vi "Get 1D Array Double Complex.vi"(5 "use temporary file? (F)":bool, 7 "data type of variable":cdb[](array[numeric]), 8 "error in":errorcluster, 10 "variable name":string, 11 "GOLPI ref. in":T1={"pipe handle"={"lv_proc.dll file path"=path "", "process instance handle"=[], "debug mode"=FALSE, "debug data"=[]}, "fast read timeout [ms]"=500, "fast read settle time [ms]"=10, "fast read to multiple [ms]"=1, "max elements per input line"=100, "slow read timeout [ms]"=5000, "stdin double format specifier"="%_16e", "max elements per stdout output column"=100, "console mode bitstream"=FALSE, "bitstream first read timeout [ms]"=1000, "bitstream read timeout [ms]"=50, "struct transfer possible"=FALSE, "matlab mode"=FALSE, "var pipe write timeout [ms]"=5000, "variable pipe mode"=FALSE, "variable pipe buffer size [Bytes]"=10000000, "variable pipe block size [Bytes]"=1000000} {"variable pipe block size [Bytes]" format="%.0p"; "variable pipe buffer size [Bytes]" format="%.0p"}) -> (0 "error out":errorcluster, 2 "value":cdb[](array[numeric]) format="%.2f", 3 "GOLPI ref. out":T1={"pipe handle"={"lv_proc.dll file path"=path "", "process instance handle"=[], "debug mode"=FALSE, "debug data"=[]}, "fast read timeout [ms]"=500, "fast read settle time [ms]"=10, "fast read to multiple [ms]"=1, "max elements per input line"=100, "slow read timeout [ms]"=5000, "stdin double format specifier"="%_16e", "max elements per stdout output column"=100, "console mode bitstream"=FALSE, "bitstream first read timeout [ms]"=1000, "bitstream read timeout [ms]"=50, "struct transfer possible"=FALSE, "matlab mode"=FALSE, "var pipe write timeout [ms]"=5000, "variable pipe mode"=FALSE, "variable pipe buffer size [Bytes]"=10000000, "variable pipe block size [Bytes]"=1000000} {"variable pipe block size [Bytes]" format="%.0p"; "variable pipe buffer size [Bytes]" format="%.0p"})   [LabVIEW 2020, in "GOLPI library.lvlib"]
doc: "Part of polymorph Get Variable.vi"
uses:
  GOLPI library.lvlib
  Public/GOLPI reference Type Def.ctl
  LV Process source distribution/Pipe Handle.ctl
  Type Definitions/Bitstream Data Type.ctl
  Type Definitions/Custom Error Codes Enum Type Def.vi
  LV Process source distribution/LV Process library.lvlib
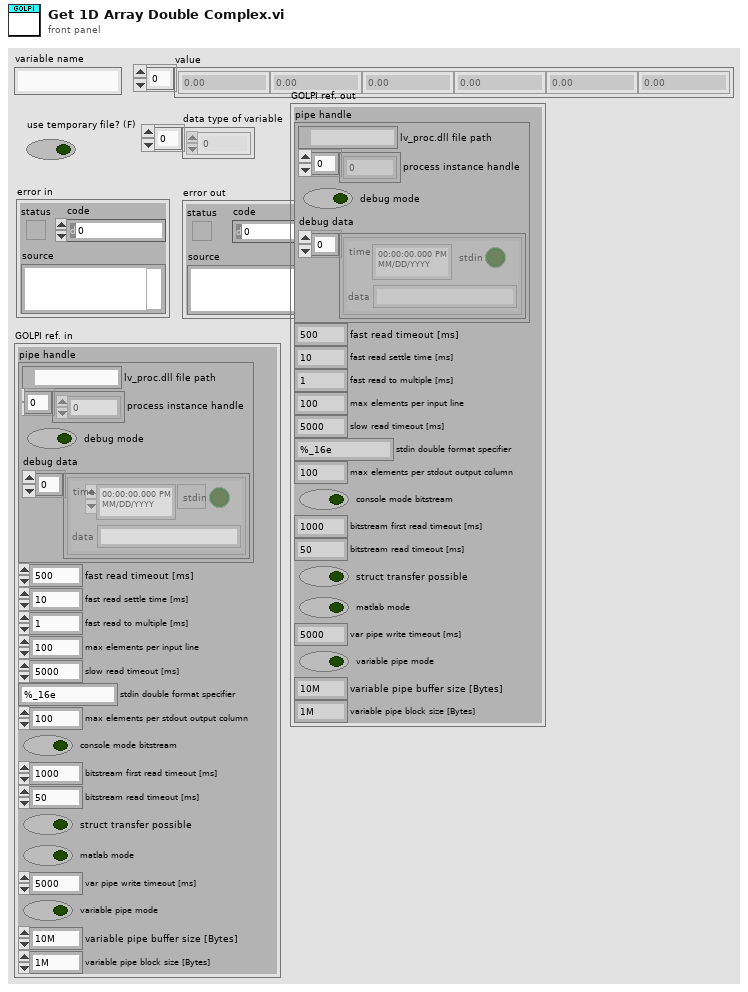
[diagram p1: front panel]
types:
  T1 = typedef "GOLPI library.lvlib/GOLPI reference Type Def.ctl" = cluster{"pipe handle":T2, "fast read timeout [ms]":u32, "fast read settle time [ms]":u32, "fast read to multiple [ms]":u32, "max elements per input line":u32, "slow read timeout [ms]":u32, "stdin double format specifier":string, "max elements per stdout output column":u32, "console mode bitstream":bool, "bitstream first read timeout [ms]":u32, "bitstream read timeout [ms]":u32, "struct transfer possible":bool, "matlab mode":bool, "var pipe write timeout [ms]":u32, "variable pipe mode":bool, "variable pipe buffer size [Bytes]":u32, "variable pipe block size [Bytes]":u32}
  T2 = typedef "LV Process library.lvlib/Pipe Handle.ctl" = cluster{"lv_proc.dll file path":path, "process instance handle":u32[], "debug mode":bool, "debug data":cluster{"time":timestamp, "stdin":bool, "data":string}[]}
  T3 = typedef "GOLPI library.lvlib/Custom Error Codes Enum Type Def.vi" = enum16{"no error", "00 working directory PAR1 missing", "01 octave binary PAR1 missing", "02 octave report error PAR1", "03 empty output last cmd PAR1", "04 missing temporary file PAR1", "05 pwd PAR 1 not exist", "06 oct package not installed", "07 octave default binary missing", "10 var PAR1 not string, vect", "11 var PAR1 not num, scal, ~compl", "12 var PAR1 not num, scal, compl", "13 var PAR1 not num, vect, ~compl", "14 var PAR1 not num, vect, compl", "15 var PAR1 not num, mat, ~compl", "16 var PAR1 not num, mat, ~compl", "30 read timeout", "60 bitstream transport failed", "61 bitstream decode error PAR1", "62 bitstream cannot be set", "70 struct transfer not possible", "80 struct: cluster elem. PAR1 not implem.", "81 struct: structure field PAR1 not implem.", "82 struct: size mismatch of PAR1", "83 struct: type mismatch of PAR1", "98 internal error", "99 not finished", "90 Not supported in Matlab mode", "91 Matlab variable transfer error", "92 Matlab Script Error"}
  T4 = typedef "GOLPI library.lvlib/Bitstream Data Type.ctl" = enum16{"dummy", "int", "uint", "float", "complex", "str", "real numeric"}
  T5 = typedef "GOLPI library.lvlib/Transfer Mode.ctl" = enum16{"Matlab", "stdio", "temp file", "bitstream", "pipe"}
  T6 = typedef "GOLPI library.lvlib/Bitstream Data.ctl" = cluster{"double":dbl[][], "cplx double":cdb[][], "int64":i64[][], "uint64":u64[][], "str":string[], "data type":T4}
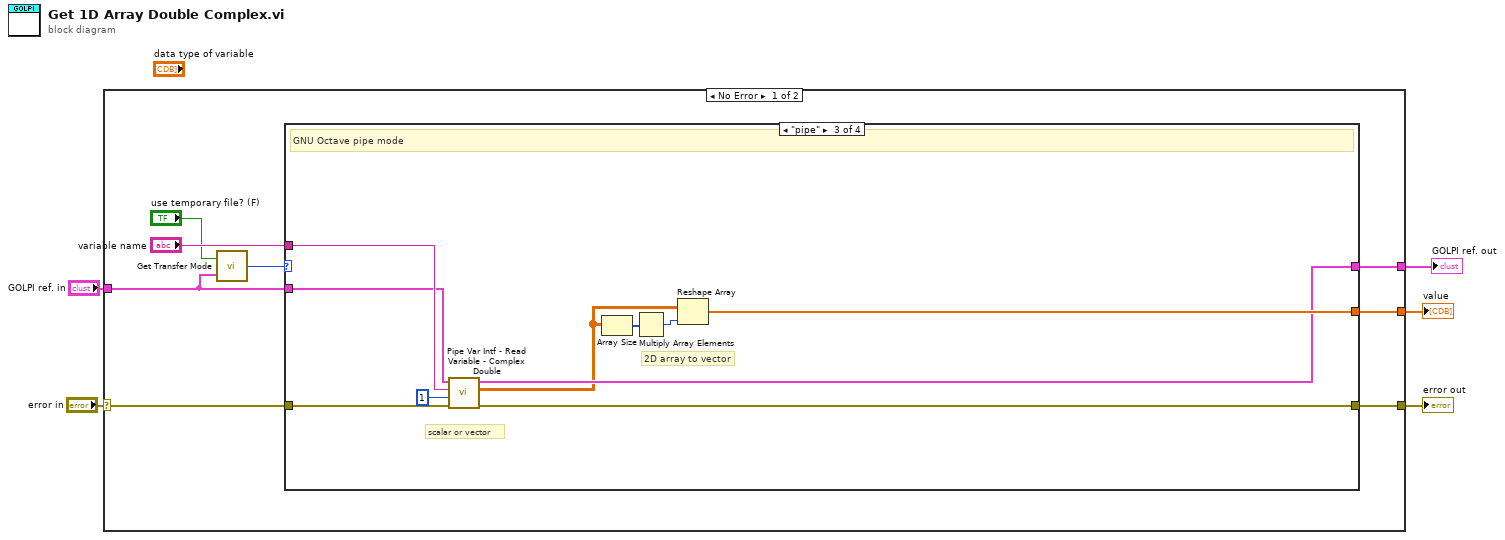
[diagram p0: block diagram]
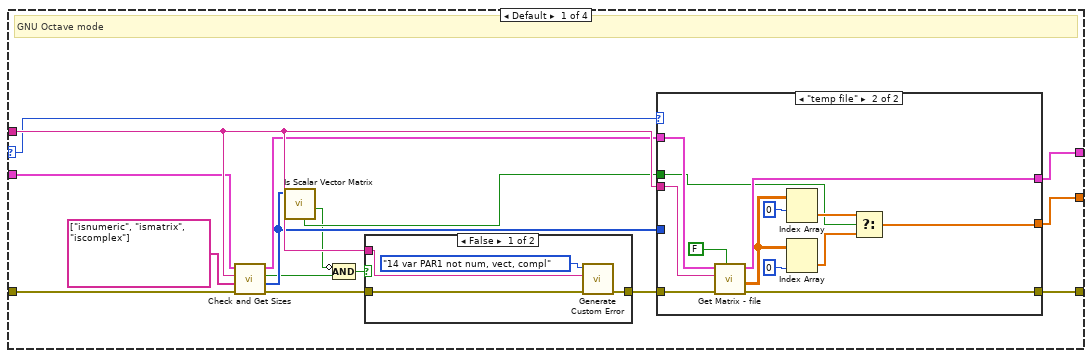
[diagram p2: hidden frame]
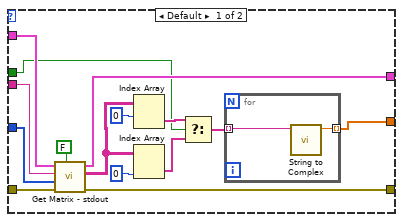
[diagram p3: hidden frame]
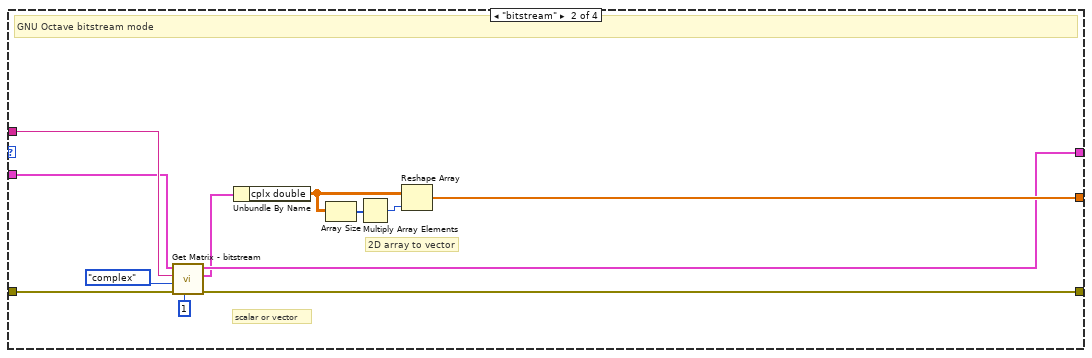
[diagram p5: hidden frame]
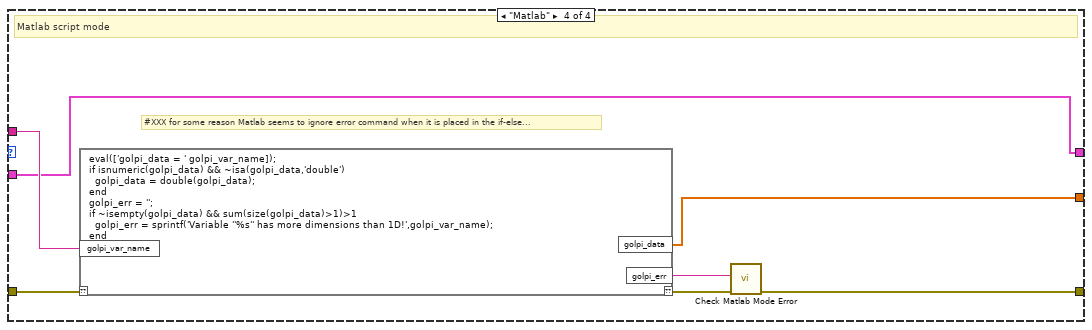
[diagram p6: hidden frame]
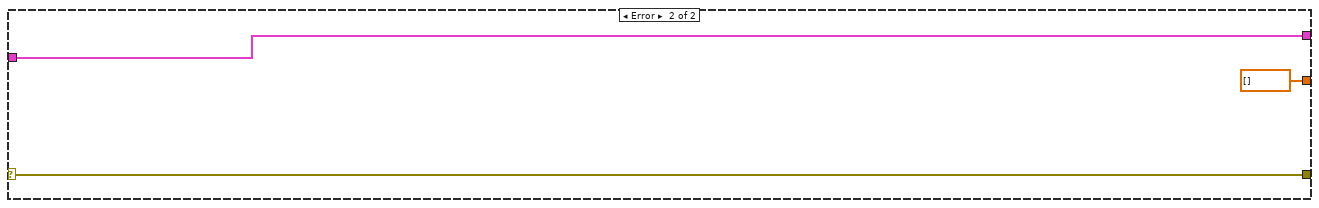
[diagram p7: hidden frame]
diagram:
  n1 = case shown="No Error" "error in" {
    selector: "error in" -> [w13 w96]
    tunnel: [w12 w96] -> w5
    tunnel: [w10 cdb[] [] ("value")] -> w3
    tunnel: "GOLPI ref. in" -> [w8 w94]
    tunnel: [w9 w94] -> w1
    frame No Error {
      n2 = call "Get Transfer Mode.vi"("GOLPI ref."=w8, "use temporary file? (F)"="use temporary file? (F)") -> ("mode"=w6:T5)
      n3 = case shown="\"pipe\"" w6 {
        selector: w6 -> [w14 _ _ _]
        tunnel: w13 -> [w29 w76 w86 w93]
        tunnel: [w28 w75 w85 w87] -> w12
        tunnel: "variable name" -> [w27 w74 w84 w92]
        tunnel: [w26 w73 w83 w90] -> w10
        tunnel: [w25 w72 w82 w91] -> w9
        tunnel: w8 -> [w24 w71 w81 w91]
        frame Default {
          # "GNU Octave mode"
          n4 = call "Check and Get Sizes.vi"("error in (no error)"=w29, "test commands"=string[] ["isnumeric", "ismatrix", "iscomplex"], "variable name"=w27, "GOLPI ref. in"=w24) -> ("error out"=w23:errorcluster, "octave sizes"=w19:i32[], "all tests OK?"=w17:bool, "GOLPI ref. out"=w21:T1)  [unwired: 4 in]
          n5 = call "Is Scalar Vector Matrix.vi"("octave sizes"=w19) -> ("is matrix?"=w15:bool, "row vector?"=w18:bool)  [unwired: 5 in, 4 out]
          n6 = Compound Arithmetic op=AND(invert w15, w17) -> (w16:bool)
          n7 = case shown="False" w16 {
            tunnel: w23 -> [w62 w64]
            tunnel: [w61 w64] -> w20
            tunnel: w27 -> [w60 _]
            frame False {
              n8 = call "Generate Custom Error.vi"("error in"=w62, "PAR1"=w60, "GOLPI error"=Custom_Error_Codes_Enum_Type_Def.vi."14 var PAR1 not num, vect, compl" ("Enum")) -> ("error out"=w61:errorcluster)  [unwired: 8 in]
            }
            frame True {
            }
          }
          n9 = case shown="\"temp file\"" w14 {
            tunnel: w21 -> [w44 w51]
            tunnel: [w43 w52] -> w25
            tunnel: w20 -> [w41 w54]
            tunnel: [w42 w53] -> w28
            tunnel: w19 -> [w40 _]
            tunnel: w18 -> [w30 w47]
            tunnel: w27 -> [w39 w48]
            tunnel: [w37 w49] -> w26
            frame Default {
              n10 = call "Get Matrix - stdout.vi"("is string?"=FALSE ("is string"), "error in (no error)"=w41, "octave sizes"=w40, "variable name"=w39, "GOLPI ref. in"=w44) -> ("error out"=w42:errorcluster, "array"=w31:string[][], "GOLPI ref. out"=w43:T1)  [unwired: 4 in]
              n11 = Index Array(array=w31, index (row)=0) -> (element=w34:string[])  [unwired: 1 in]
              n12 = Index Array(array=w31, index (col)=0 ("disabled index (col)")) -> (element=w33:string[])  [unwired: 1 in]
              n13 = Select(t=w34, s=w30, f=w33) -> (s? t:f=w32:string[])
              n14 = for {
                tunnel: w32 -> [w46] mode=indexing
                tunnel: [w45] -> w37 mode=indexing
                n15 = call "String to Complex.vi"("string"=w46) -> ("complex number"=w45:cdb)  [unwired: 10 in]
              }
            }
            frame "temp file" {
              n16 = call "Get Matrix - file.vi"("is string?"=FALSE ("is string"), "error in (no error)"=w54, "variable name"=w48, "GOLPI ref. in"=w51) -> ("error out"=w53:errorcluster, "cmplx double array"=w50:cdb[][], "GOLPI ref. out"=w52:T1)  [unwired: 3 in, 2 out]
              n17 = Index Array(array=w50, index (row)=0) -> (element=w57:cdb[])  [unwired: 1 in]
              n18 = Index Array(array=w50, index (col)=0 ("disabled index (col)")) -> (element=w56:cdb[])  [unwired: 1 in]
              n19 = Select(t=w57, s=w47, f=w56) -> (s? t:f=w49:cdb[])
            }
          }
        }
        frame "bitstream" {
          # "scalar or vector"
          # "2D array to vector"
          # "GNU Octave bitstream mode"
          n20 = call "Get Matrix - bitstream.vi"("max dimensions (0: scalar)"=1, "error in (no error)"=w76, "data type"=Bitstream_Data_Type."complex", "variable name"=w74, "GOLPI ref. in"=w71) -> ("error out"=w75:errorcluster, "data"=w65:T6, "GOLPI ref. out"=w72:T1)  [unwired: 4 in]
          n21 = Unbundle By Name(w65) -> ("cplx double"=w68:cdb[][])
          n22 = Array Size(array=w68) -> (size(s)=w67:i32[])
          n23 = Multiply Array Elements(1:w67) -> (0:w66:i32)
          n24 = Reshape Array(w68, w66) -> (w73:cdb[])
        }
        frame "pipe" {
          # "scalar or vector"
          # "2D array to vector"
          # "GNU Octave pipe mode"
          n25 = call "Pipe Var Intf - Read Variable - Complex Double.vi"("error in (no error)"=w86, "max dims (0: scalar)"=1 ("max dimensions (0: scalar)"), "variable name"=w84, "GOLPI ref. in"=w81) -> ("error out"=w85:errorcluster, "data out"=w77:cdb[][], "GOLPI ref. out"=w82:T1)  [unwired: 5 in]
          n26 = Array Size(array=w77) -> (size(s)=w79:i32[])
          n27 = Multiply Array Elements(1:w79) -> (0:w78:i32)
          n28 = Reshape Array(w77, w78) -> (w83:cdb[])
        }
        frame "Matlab" {
          # "#XXX for some reason Matlab seems to ignore error command when it is placed in the if-else..."
          # "Matlab script mode"
          n29 = script code="eval(['golpi_data = ' golpi_var_name]);\nif isnumeric(golpi_data) && ~isa(golpi_data,'double')\n  golpi_data = double(golpi_data);\nend\ngolpi_err = '';\nif ~isempty(golpi_data) && sum(size(golpi_data)>1)>1\n  golpi_err = sprintf('Variable ''%s'' has more dimensions than 1D!',golpi_var_name);\nend"("??"=w93, "golpi_var_name"=w92) -> ("??"=w89:errorcluster, "golpi_data"=w90:cdb[], "golpi_err"=w88:string)
          n30 = call "Check Matlab Mode Error.vi"("error in"=w89, "custom error string (empty)"=w88) -> ("error out"=w87:errorcluster)  [unwired: 9 in]
        }
      }
    }
    frame Error {
    }
  }
  "value" <- w3
  "error out" <- w5
  "GOLPI ref. out" <- w1
